vi "Splash Screen.vi"   [LabVIEW 2013, in "Listener Launcher.lvlib"]
doc: "This is the top-level VI of this application. When it runs, it behaves like the splash screen many applications use to keep the user occupied while the application loads into memory. This application is quite small, so there is little overhead, which would make the splash screen just flash for a moment. Because that flash is distracting, there is a three-second delay inserted into this VI so that it stays up for a little bit. \n\nThis VI uses a delay-loaded subVI call to load the rest of the application. This trick ensures that the splash screen can load instantly regardless of how large the rest of the VI hierarchy gets, and the loading of the rest of the VIs becomes one step in the load process."
uses:
  Listener Launcher.lvlib
  LVAutomationListener/LVAutomationListener/Load App.vi
  LVAutomationListener/LVAutomationListener/LVAutomationListener.lvclass
panel:
  # "Loading LabVIEW Listener..."
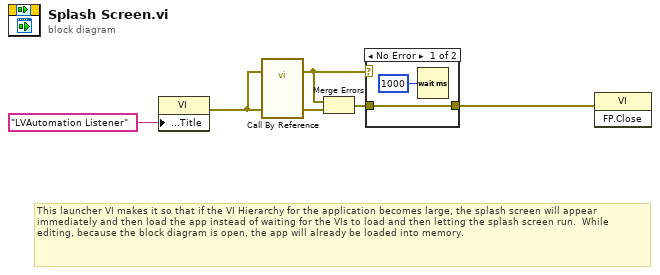
[diagram p0: block diagram]
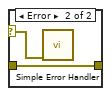
[diagram p2: hidden frame]
diagram:
  # "This launcher VI makes it so that if the VI Hierarchy for the application becomes large, the splash screen will appear immediately and then load the app instead of waiting for the VIs to load and then letting the splash screen run.  While editing, because the block diagram is open, the app will already be loaded into memory."
  n1 = property class="VI"("Front Panel.Title"="LVAutomation Listener" ("Window Title")) -> (error out=w2:errorcluster)  [unwired: 2 in, 1 out]
  n2 = call-by-ref "?"(error in=w2, 8:"error in (no error)"=w2) -> (error out=w4:errorcluster, 0:"error out"=w6:errorcluster)  [unwired: 11 in, 1 out]
  n3 = Merge Errors(w4, w6) -> (w5:errorcluster)
  n4 = case shown="No Error" w4 {
    tunnel: [w8 w9] -> w1
    tunnel: w5 -> [w8 w9]
    selector: w4 -> [_ w10]
    frame No Error {
      n5 = Wait (ms)(milliseconds to wait=u32 1000) -> ()  [unwired: 1 out]
    }
    frame Error {
      n6 = call <vilib>:"Simple Error Handler.vi"("error in (no error)"=w10) -> ()  [unwired: 4 in, 5 out]
    }
  }
  n7 = invoke class="VI" method="FP.Close"(error in=w1) -> ()  [unwired: 2 in, 3 out]
